vi "DllFxpAddSub_Int.vi"(6 "cin/nbin":bool, 8 "load":bool=TRUE, 9 "is sub":bool, 10 "y":u32, 11 "x":u32) -> (2 "cout/nbout/overflow":bool, 3 "s":u32)   [LabVIEW 2017]
uses:
  <vilib>/rvi/FXPMathLib/sim/FxpSim.dll
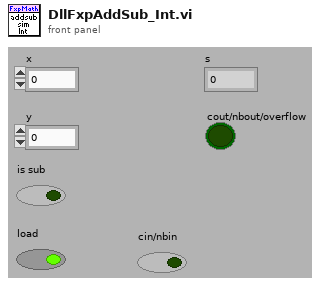
[diagram p1: front panel]
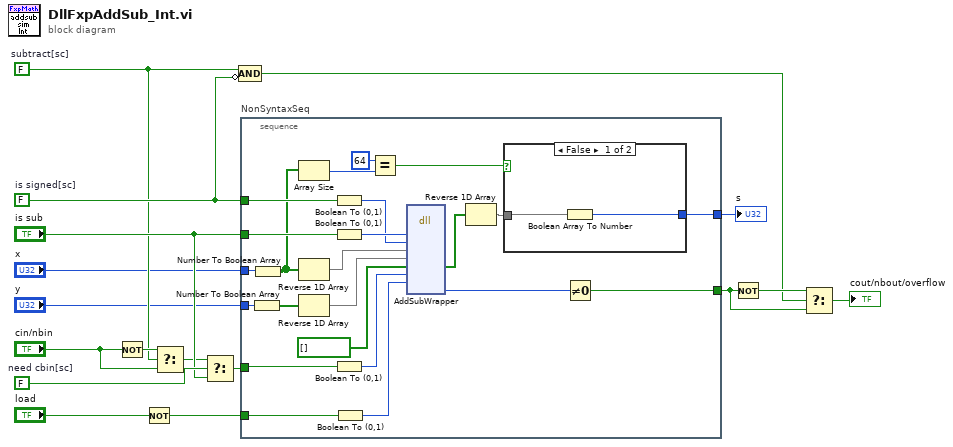
[diagram p0: block diagram]
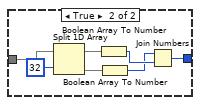
[diagram p2: hidden frame]
diagram:
  w5 = FALSE  # subtract[sc]
  w6 = FALSE  # is signed[sc]
  w17 = FALSE  # need cbin[sc]
  n1 = Not(x="cin/nbin") -> (.not. x?=w11:bool)
  n2 = Not(x="load") -> (.not. x?=w3:bool)
  n3 = Select(t=w11, s=w5, f="cin/nbin") -> (s? t:f=w12:bool)
  n4 = Select(t=w12, s=w17, f="is sub") -> (s? t:f=w16:bool)
  n5 = Compound Arithmetic op=AND(w5, invert w6) -> (w4:bool)
  n6 = stacked-sequence "NonSyntaxSeq" {
    tunnel: [w40] -> w8
    tunnel: "is sub" -> [w39]
    tunnel: w16 -> [w36]
    tunnel: w3 -> [w35]
    tunnel: w6 -> [w34]
    tunnel: [w33] -> w13
    tunnel: "x" -> [w21]
    tunnel: "y" -> [w19]
    frame #0 {
      n7 = Number To Boolean Array(number=w19) -> (Boolean array=w18:bool[])
      n8 = Number To Boolean Array(number=w21) -> (Boolean array=w20:bool[])
      n9 = Array Size(array=w20) -> (size(s)=w26:i32)
      n10 = Reverse 1D Array(array=w20) -> (reversed array=w22:bool[])
      n11 = Reverse 1D Array(array=w18) -> (reversed array=w23:bool[])
      n12 = Boolean To (0,1)(Boolean=w34) -> (0, 1=w37:i16)
      n13 = Boolean To (0,1)(Boolean=w39) -> (0, 1=w38:i16)
      n14 = Boolean To (0,1)(Boolean=w36) -> (0, 1=w29:i16)
      n15 = Boolean To (0,1)(Boolean=w35) -> (0, 1=w30:i16)
      n16 = Equal?(x=64, y=w26) -> (x = y?=w24:bool)
      n17 = dll-call lib="e:/penguin/lvdist/win32/export/17.0/17.0.1f1/dist/vi.lib/rvi/FXPMathLib/sim/FxpSim.dll" fn="AddSubWrapper"("isSub"=w38, "isSigned"=w37, "xH"=w22, "yH"=w23, "zH"=bool[] [] ("xH"), "CinOrNBin"=w29, "notLoad"=w30) -> ("zH"=w27:bool[], "CoutOrNBoutOrOvfl"=w31:u8)  [unwired: 3 in, 10 out]
      n18 = Reverse 1D Array(array=w27) -> (reversed array=w32:bool[])
      n19 = case shown="False" w24 {
        tunnel: w32 -> [w42 w49]
        tunnel: [w41 w45] -> w33
        frame False {
          n20 = Boolean Array To Number(Boolean array=w42) -> (number=w41:u32)
        }
        frame True {
          n21 = Split 1D Array(array=w49, index=32) -> (first subarray=w47:bool[], second subarray=w46:bool[])
          n22 = Boolean Array To Number(Boolean array=w47) -> (number=w44:u32)
          n23 = Boolean Array To Number(Boolean array=w46) -> (number=w43:u32)
          n24 = Join Numbers(hi=w43, lo=w44) -> ((hi.lo)=w45:u64)
        }
      }
      n25 = Not Equal To 0?(x=w31) -> (x != 0?=w40:bool)
    }
  }
  "s" <- w13
  n26 = Not(x=w8) -> (.not. x?=w9:bool)
  n27 = Select(t=w9, s=w4, f=w8) -> (s? t:f=→"cout/nbout/overflow":bool)
